vi "CAL-Compute Freefield ASTF.vi"(0 "Mag":dbl[][](array[numeric]), 1 "Stimulus":dbl[](array[numeric]), 5 "Phase":dbl[][](array[numeric]), 7 "df (Hz)":dbl, 9 "Mic Gain (dB)":dbl=50000.0, 11 "error in (no error)":errorcluster, 12 "Attenuation (dB)":dbl, 13 "Compute Options":T1={"Cal Mic Sens"=-146.12351367888365, "UseMicCal"=FALSE, "Path"=path ""} {"Cal Mic Sens" format="%.2f"}) -> (4 "ASTF Mag":dbl[](array[numeric]), 6 "ASTF Phase":dbl[](array[numeric]), 8 "Frequency":dbl[](array[numeric]), 15 "error out":errorcluster)   [LabVIEW 2015]
uses:
  Utility VIs/Math VIs/FFT x(t) to dB,Degrees (1D).vi
  Utility VIs/Math VIs/LinSpace (x0-dx-npts).vi
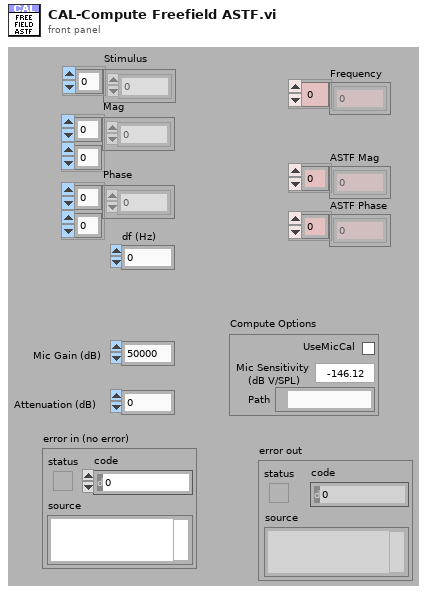
[diagram p1: front panel]
types:
  T1 = cluster{"Cal Mic Sens":dbl, "UseMicCal":bool, "Path":path}
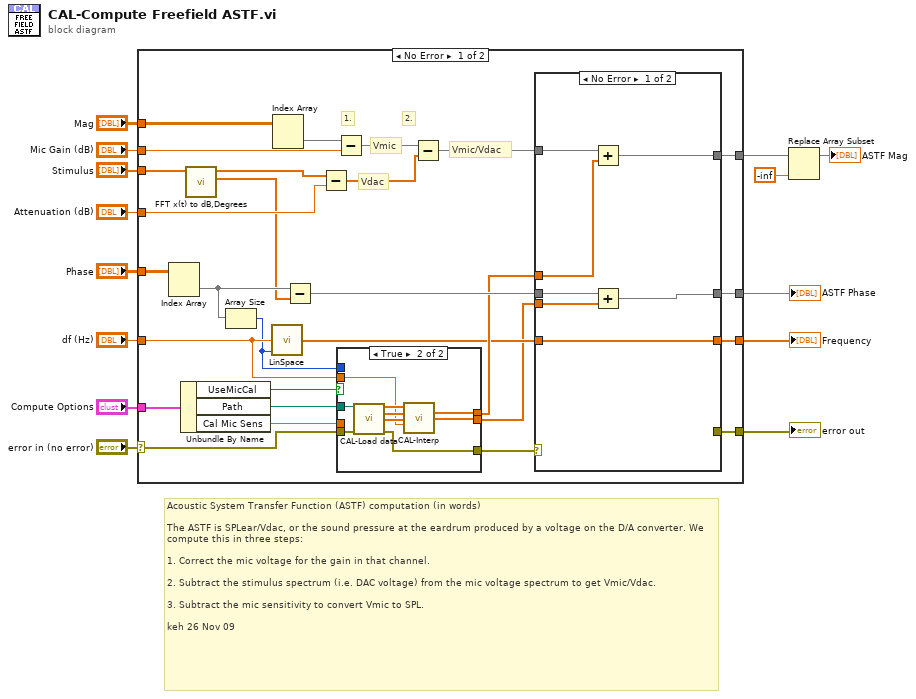
[diagram p0: block diagram]
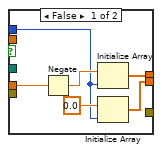
[diagram p3: hidden frame]
diagram:
  # "Acoustic System Transfer Function (ASTF) computation (in words)\n\nThe ASTF is SPLear/Vdac, or the sound pressure at the eardrum produced by a voltage on the D/A converter. We compute this in three steps:\n\n1. Correct the mic voltage for the gain in that channel.\n\n2. Subtract the stimulus spectrum (i.e. DAC voltage) from the mic voltage spectrum to get Vmic/Vdac.\n\n3. Subtract the mic sensitivity to convert Vmic to SPL.\n\nkeh 26 Nov 09"
  n1 = case shown="No Error" "error in (no error)" {
    selector: "error in (no error)" -> [w30 w66]
    tunnel: "Mag" -> [w42 _]
    tunnel: "Phase" -> [w41 _]
    tunnel: [w34 _] -> w12
    tunnel: [w24 _] -> w11
    tunnel: "Stimulus" -> [w38 _]
    tunnel: "df (Hz)" -> [w17 _]
    tunnel: [w20 _] -> w7
    tunnel: "Mic Gain (dB)" -> [w16 _]
    tunnel: [w22 w66] -> w5
    tunnel: "Attenuation (dB)" -> [w39 _]
    tunnel: "Compute Options" -> [w18 _]
    frame No Error {
      # "2."
      # "1."
      # "Vmic/Vdac"
      # "Vdac"
      # "Vmic"
      n2 = Index Array(array=w41) -> (element=w40:dbl[])  [unwired: 2 in]
      n3 = Unbundle By Name(w18) -> ("UseMicCal"=w29:bool, "Path"=w28:path, "Cal Mic Sens"=w27:dbl)
      n4 = call-poly "FFT x(t) to dB,Degrees.vi"("X"=w38) -> ("+Freq Phase of FFT (degrees)"=w37:dbl[], "+Freq. Mag of FFT (dB rms)"=w36:dbl[])  [unwired: 8 in, 1 out]
      n5 = Array Size(array=w40) -> (size(s)=w15:i32)
      n6 = call-poly "LinSpace.vi"("npts"=w15, "dx"=w17) -> ("Array"=w21:dbl[])  [unwired: 2 in, 1 out]
      n7 = Index Array(array=w42) -> (element=w33:dbl[])  [unwired: 2 in]
      n8 = Subtract(x=w40, y=w37) -> (x-y=w25:dbl[])
      n9 = Subtract(x=w36, y=w39) -> (x-y=w35:dbl[])
      n10 = Subtract(x=w33, y=w16) -> (x-y=w32:dbl[])
      n11 = case shown="True" w29 {
        tunnel: w30 -> [_ w65]
        tunnel: w28 -> [_ w64]
        tunnel: w27 -> [w56 _]
        tunnel: [_ w63] -> w26
        tunnel: [w55 w59] -> w23
        tunnel: [w52 w58] -> w19
        tunnel: w17 -> [_ w57]
        tunnel: w15 -> [w51 _]
        frame False {
          n12 = Negate(x=w56) -> (-x=w54:dbl)
          n13 = Initialize Array(w54, w51) -> (w55:dbl[])
          n14 = Initialize Array(0.0 ("element"), w51) -> (w52:dbl[])
        }
        frame True {
          n15 = call "CAL-Load data.vi"("user path"=w64, "error in (no error)"=w65) -> ("Frequency (Hz)"=w62:dbl[], "Mag"=w61:dbl[], "Phase"=w60:dbl[], "error out"=w63:errorcluster)  [unwired: 6 in, 4 out]
          n16 = call "CAL-Interp.vi"("Frequency (Hz)"=w62, "Magnitude (dB)"=w61, "Phase (degrees)"=w60, "df (Hz)"=w57) -> ("Interp Magnitude (dB)"=w59:dbl[], "Interp Phase (degrees)"=w58:dbl[])  [unwired: 8 in, 2 out]
        }
      }
      n17 = Subtract(x=w32, y=w35) -> (x-y=w31:dbl[])
      n18 = case shown="No Error" w26 {
        selector: w26 -> [_ w50]
        tunnel: w23 -> [w49 _]
        tunnel: [w48 _] -> w34
        tunnel: w31 -> [w47 _]
        tunnel: [_ w50] -> w22
        tunnel: w25 -> [w46 _]
        tunnel: [w45 _] -> w24
        tunnel: w21 -> [w44 _]
        tunnel: [w44 _] -> w20
        tunnel: w19 -> [w43 _]
        frame No Error {
          n19 = Add(x=w47, y=w49) -> (x+y=w48:dbl[])
          n20 = Add(x=w46, y=w43) -> (x+y=w45:dbl[])
        }
        frame Error {
        }
      }
    }
    frame Error {
    }
  }
  "ASTF Phase" <- w11
  "error out" <- w5
  "Frequency" <- w7
  n21 = Replace Array Subset(array=w12, new element=-inf) -> (→"ASTF Mag":dbl[])  [unwired: 1 in]
